vi "Is Sub-Section of.vi"(8 "error in":errorcluster, 10 "Parent Section Name":refnum<class "Section Name.lvclass">, 11 "Section Name in":refnum<class "Section Name.lvclass">) -> (0 "error out":errorcluster, 2 "Is Sub-Section of?":bool, 3 "Section Name out":refnum<class "Section Name.lvclass">)   [LabVIEW 2024, in "Electronic Datasheet.lvlib" / "Section Name.lvclass"]
uses:
  Section Name.lvclass
  Section Name.lvclass/Section Name.ctl
  <vilib>/regexp/Match Regular Expression.xnode
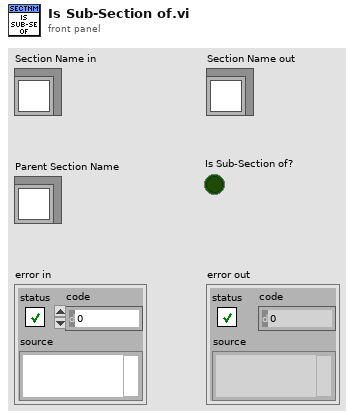
[diagram p1: front panel]
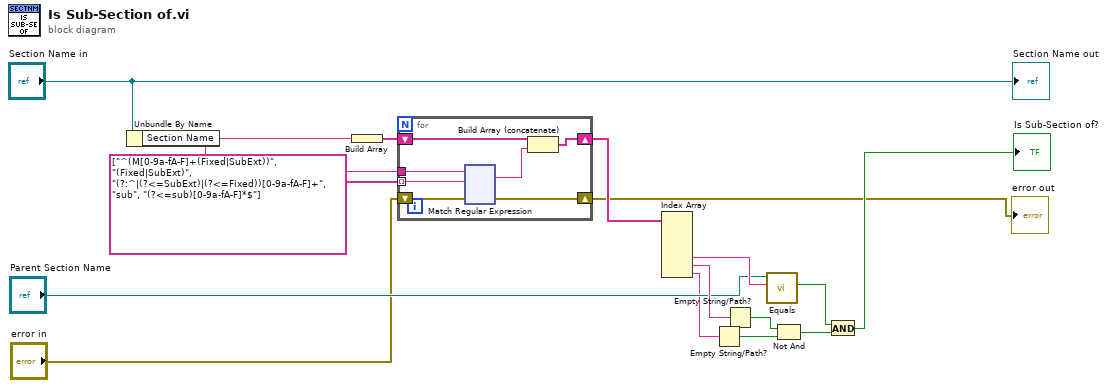
[diagram p0: block diagram]
diagram:
  n1 = Unbundle By Name("Section Name in") -> ("Section Name"=w11:string)
  n2 = Build Array(w11) -> (w16:string[])
  n3 = for {
    tunnel: string[] ["^(M[0-9a-fA-F]+(Fixed|SubExt))", "(Fixed|SubExt)", "(?:^|(?<=SubExt)|(?<=Fixed))[0-9a-fA-F]+", "sub", "(?<=sub)[0-9a-fA-F]*$"] -> [w23] mode=indexing
    shift-right: [w21] -> w14
    shift-left: w16 -> [w22]
    tunnel: w11 -> [w19]
    shift-right: [w17] -> w1
    shift-left: "error in" -> [w18]
    n4 = xnode "Match Regular Expression"("input string"=w19, "regular expression"=w23, "error in"=w18) -> ("whole match"=w20:string, "error out"=w17:errorcluster)  [unwired: 3 in, 3 out]
    n5 = Build Array (concatenate)(w22, w20) -> (w21:string[])
  }
  "error out" <- w1
  n6 = Index Array(array=w14) -> (element #4=w9:string, element #5=w12:string, element #6=w7:string)  [unwired: 6 in, 3 out]
  n7 = Empty String/Path?(string/path=w7) -> (empty?=w6:bool)
  n8 = Empty String/Path?(string/path=w12) -> (empty?=w13:bool)
  n9 = call "Equals.vi"("String"=w9, "Section Name in"="Parent Section Name") -> ("Equal?"=w3:bool)  [unwired: 8 in, 1 out]
  n10 = Not And(1:w6, 2:w13) -> (0:w5:bool)
  n11 = And(x=w3, y=w5) -> (x .and. y?=→"Is Sub-Section of?":bool)
  "Section Name out" <- "Section Name in"
